vi "Unregister and Close Sessions.vi"(8 "error in":errorcluster) -> (0 "error out":errorcluster)   [LabVIEW 2021, in "SourceMeasureDCVoltage.lvlib"]
uses:
  SourceMeasureDCVoltage.lvlib
  <vilib>/Plug-In SDKs/Clients/Session Management V1/Session Reservation/Session Reservation.lvclass/Session Reservation.ctl
  FAL/Instruments/Abstract_Instrument/controls/Initialize_Info.ctl
  <vilib>/Plug-In SDKs/Clients/Session Management V1/Session Reservation/Initialize and Close Session Behavior.ctl
  <vilib>/Plug-In SDKs/Clients/Session Management V1/Session Reservation/Merge Invalid DVR Error.vi
  <vilib>/Plug-In SDKs/Clients/Session Management V1/Session Reservation/Is DVR Valid.vi
  <vilib>/Plug-In SDKs/Measurements/Helpers/Error Strings Global Internal.vi
  <vilib>/Utility/error.llb/Error Cluster From Error Code.vi
  FAL/Instruments/Abstract_Instrument/Abstract_Instrument.lvclass
  <vilib>/Plug-In SDKs/Clients/Session Management V1/Session Reservation/Session Reservation.lvclass
  FAL/Reusables/Get Pin Information.lvlib
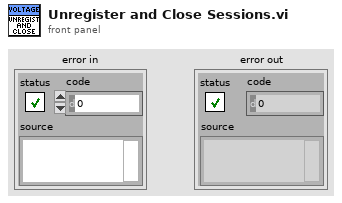
[diagram p1: front panel]
types:
  T1 = typedef "Abstract_Instrument.lvclass/Initialize_Info.ctl" = cluster{"initialize and close session behavior":T2, "reset":bool, "optional string":string}
  T2 = typedef "NI Session Management V1 Client.lvlib/Session Reservation.lvclass/Initialize and Close Session Behavior.ctl" = enum16{"Auto", "Initialize and Close", "Attach and Detach", "Initialize and Detach", "Attach and Close"}
  T3 = typedef "ni.measurementlink.sessionmanagement.v1.api.lvlib/ni_measurementlink_sessionmanagement_v1_SessionInformation.ctl" = cluster{"session":T4, "resource_name":string, "channel_list":string, "instrument_type_id":string, "session_exists":bool, "channel_mappings":T5[]}
  T4 = typedef "ni.measurementlink.sessionmanagement.v1.api.lvlib/nidevice_grpc_Session.ctl" = cluster{"name":string}
  T5 = typedef "ni.measurementlink.sessionmanagement.v1.api.lvlib/ni_measurementlink_sessionmanagement_v1_ChannelMapping.ctl" = cluster{"pin_or_relay_name":string, "site":i32, "channel":string, "multiplexer_resource_name":string, "multiplexer_route":string}
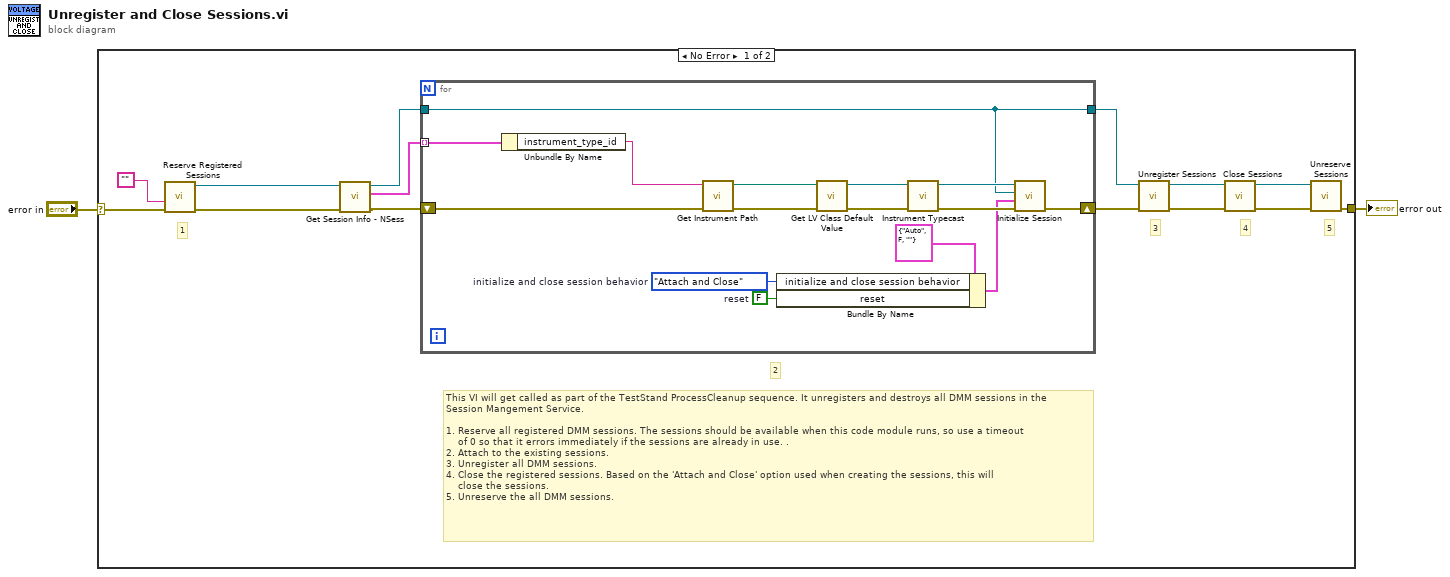
[diagram p0: block diagram]
diagram:
  n1 = case shown="No Error" "error in" {
    selector: "error in" -> [w16 w32]
    tunnel: [w3 w32] -> w1
    frame No Error {
      # "5"
      # "4"
      # "3"
      # "2"
      # "1"
      # "This VI will get called as part of the TestStand ProcessCleanup sequence. It unregisters and destroys all DMM sessions in the\nSession Mangement Service.\n\n1. Reserve all registered DMM sessions. The sessions should be available when this code module runs, so use a timeout\n    of 0 so that it errors immediately if the sessions are already in use. .\n2. Attach to the existing sessions.\n3. Unregister all DMM sessions.\n4. Close the registered sessions. Based on the 'Attach and Close' option used when creating the sessions, this will\n    close the sessions.\n5. Unreserve the all DMM sessions."
      n2 = call <vilib>:"Reserve Registered Sessions.vi"("error in"=w16, "instrument type id"="") -> ("error out"=w12:errorcluster, "session reservation out"=w11:refnum<class "Session Reservation.lvclass">)  [unwired: 8 in]
      n3 = call <vilib>:"Get Session Info - NSess .vi"("error in"=w12, "session reservation in"=w11) -> ("error out"=w15:errorcluster, "sessions info"=w14:T3[], "session reservation out"=w13:refnum<class "Session Reservation.lvclass">)  [unwired: 7 in]
      n4 = for {
        shift-right: [w27] -> w7
        shift-left: w15 -> [w17]
        tunnel: w14 -> [w31] mode=indexing
        tunnel: w13 -> [w22]
        tunnel: [w22] -> w6
        w21 = Initialize_and_Close_Session_Behavior."Attach and Close"  # initialize and close session behavior
        w23 = FALSE  # reset
        n5 = Unbundle By Name(w31) -> ("instrument_type_id"=w20:string)
        n6 = call "Get Instrument Path.vi"("error in"=w17, "instrument_type_id"=w20) -> ("error out"=w18:errorcluster, "Instrument Path"=w19:path)  [unwired: 8 in]
        n7 = Bundle By Name(cluster=T1 {"initialize and close session behavior"=enum."Auto", "reset"=FALSE, "optional string"=""} ("Initialize_Info"), "initialize and close session behavior"=w21, "reset"=w23) -> (w24:T1)
        n8 = call <vilib>:"Get LV Class Default Value.vi"("error in (no error)"=w18, "class path"=w19) -> ("error out"=w30:errorcluster, "object"=w29:refnum<class>)  [unwired: 8 in]
        n9 = call "Instrument Typecast.vi"("error in (no error)"=w30, "pin instrument"=w29) -> ("error out"=w28:errorcluster, "instrument object"=w26:refnum<class "Abstract_Instrument.lvclass">)  [unwired: 8 in]
        n10 = call-dynamic "Initialize Session.vi"("error in (no error)"=w28, "Initialize_Info"=w24, "session reservation in"=w22, "Abstract_Instrument in"=w26) -> ("error out"=w27:errorcluster)  [unwired: 6 in, 1 out]
      }
      n11 = call <vilib>:"Unregister Sessions.vi"("error in"=w7, "session reservation in"=w6) -> ("error out"=w8:errorcluster, "session reservation out"=w5:refnum<class "Session Reservation.lvclass">)  [unwired: 8 in]
      n12 = call <vilib>:"Close Sessions.vi"("error in"=w8, "session reservation in"=w5) -> ("error out"=w9:errorcluster, "session reservation out"=w4:refnum<class "Session Reservation.lvclass">)  [unwired: 8 in]
      n13 = call <vilib>:"Unreserve Sessions.vi"("error in"=w9, "session reservation in"=w4) -> ("error out"=w3:errorcluster)  [unwired: 9 in]
    }
    frame Error {
    }
  }
  "error out" <- w1
